vi "Compile Steps.vi"(8 "error in (no error)":errorcluster, 11 "Plugin in":refnum<class "Output Sequencer.lvclass">) -> (0 "error out":errorcluster, 3 "Plugin out":refnum<class "Output Sequencer.lvclass">)   [LabVIEW 2024, in "Output Sequencer.lvlib" / "Output Sequencer.lvclass"]
uses:
  Output Sequencer.lvclass
  Output Sequencer.lvclass/Output Sequencer.ctl
  Types/Expression Data.ctl
  <vilib>/LAVA/muParser/mupExpr/mupExpr.lvclass
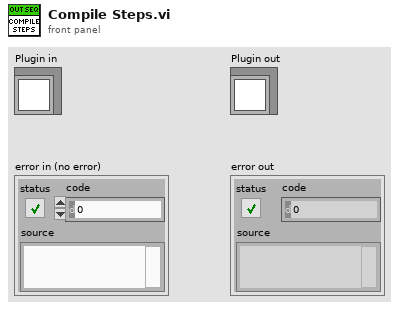
[diagram p1: front panel]
types:
  T1 = typedef "Output Sequencer.lvlib/Output Sequencer.lvclass/Expression Data.ctl" = cluster{"Empty?":bool, "Expression":refnum<class "mupExpr.lvclass">, "Variable Names":string[]}
  T2 = typedef "Output Sequencer.lvlib/Settings UI.lvclass/Step Settings.ctl" = cluster{"Description":string, "Precondition":string, "Duration":dbl, "Mode":string, "Delay Between Values":dbl, "Analog Values":string[], "Digital Values":string[], "Postcondition":string, "On True":string, "On False":string}
  T3 = typedef "Output Sequencer.lvlib/Output Sequencer.lvclass/Compiled Step.ctl" = cluster{"Precondition":T1, "Duration":dbl, "Mode":string, "Delay Between Values":dbl, "Analog Values":T1[], "Digital Values":T1[], "Postcondition":T1, "On True":string, "On False":string}
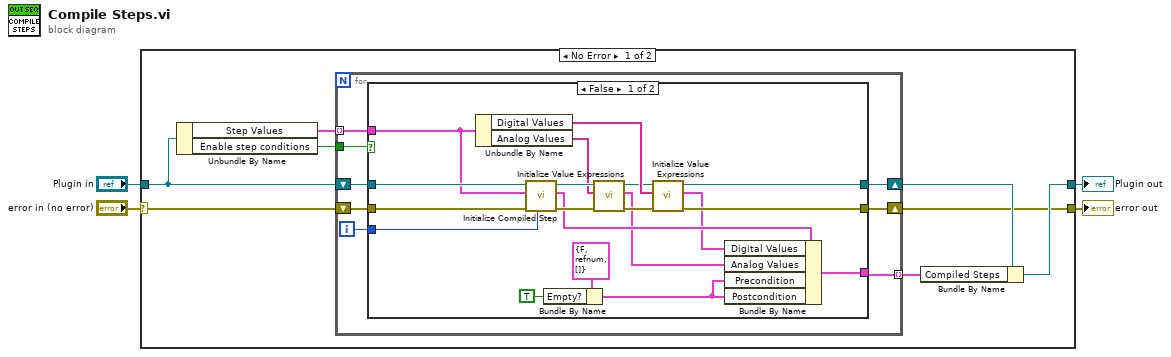
[diagram p0: block diagram]
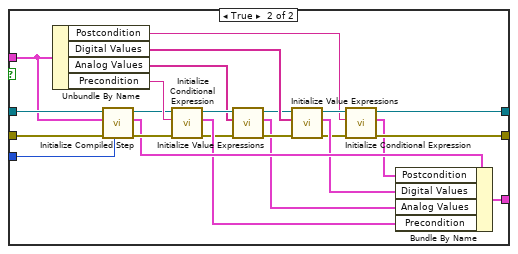
[diagram p2: hidden frame]
diagram:
  n1 = case shown="No Error" "error in (no error)" {
    selector: "error in (no error)" -> [w5 w65]
    tunnel: [w10 w64] -> w4
    tunnel: [w8 w65] -> w3
    tunnel: "Plugin in" -> [w7 w64]
    frame No Error {
      n2 = Unbundle By Name(w7) -> ("Step Values"=w12:T2[], "Enable step conditions"=w6:bool)
      n3 = for {
        tunnel: w12 -> [w18] mode=indexing
        tunnel: [w16] -> w11 mode=indexing
        shift-right: [w15] -> w9
        shift-left: w7 -> [w20]
        shift-right: [w17] -> w8
        shift-left: w5 -> [w19]
        tunnel: w6 -> [w14]
        i -> [w13]
        n4 = case shown="False" w14 {
          tunnel: w20 -> [w39 w63]
          tunnel: w19 -> [w38 w62]
          tunnel: w18 -> [w37 w61]
          tunnel: [w34 w57] -> w17
          tunnel: [w32 w53] -> w16
          tunnel: [w25 w42] -> w15
          tunnel: w13 -> [w21 w40]
          frame False {
            n5 = Unbundle By Name(w37) -> ("Digital Values"=w30:string[], "Analog Values"=w31:string[])
            n6 = call "Initialize Compiled Step.vi"("Step Number"=w21, "error in (no error)"=w38, "Step Values"=w37, "Output Sequencer in"=w39) -> ("error out"=w36:errorcluster, "Compiled Step"=w33:T3, "Output Sequencer out"=w35:refnum<class "Output Sequencer.lvclass">)  [unwired: 5 in]
            n7 = Bundle By Name(cluster=T1 {"Empty?"=FALSE, "Expression"=refnum, "Variable Names"=[]} ("Precondition"), "Empty?"=TRUE) -> (w22:T1)
            n8 = call "Initialize Value Expressions.vi"("error in (no error)"=w36, "Value strings"=w31, "Output Sequencer in"=w35) -> ("error out"=w28:errorcluster, "Expressions"=w27:T1[], "Output Sequencer out"=w29:refnum<class "Output Sequencer.lvclass">)  [unwired: 6 in]
            n9 = call "Initialize Value Expressions.vi"("error in (no error)"=w28, "Value strings"=w30, "Output Sequencer in"=w29) -> ("error out"=w34:errorcluster, "Expressions"=w26:T1[], "Output Sequencer out"=w25:refnum<class "Output Sequencer.lvclass">)  [unwired: 6 in]
            n10 = Bundle By Name(cluster=w33, "Digital Values"=w26, "Analog Values"=w27, "Precondition"=w22, "Postcondition"=w22) -> (w32:T3)
          }
          frame True {
            n11 = Unbundle By Name(w61) -> ("Postcondition"=w41:string, "Digital Values"=w49:string[], "Analog Values"=w50:string[], "Precondition"=w59:string)
            n12 = call "Initialize Compiled Step.vi"("Step Number"=w40, "error in (no error)"=w62, "Step Values"=w61, "Output Sequencer in"=w63) -> ("error out"=w60:errorcluster, "Compiled Step"=w56:T3, "Output Sequencer out"=w58:refnum<class "Output Sequencer.lvclass">)  [unwired: 5 in]
            n13 = call "Initialize Conditional Expression.vi"("error in (no error)"=w60, "Expression string"=w59, "Output Sequencer in"=w58) -> ("error out"=w51:errorcluster, "Expression Data"=w55:T1, "Output Sequencer out"=w52:refnum<class "Output Sequencer.lvclass">)  [unwired: 6 in]
            n14 = call "Initialize Value Expressions.vi"("error in (no error)"=w51, "Value strings"=w50, "Output Sequencer in"=w52) -> ("error out"=w47:errorcluster, "Expressions"=w46:T1[], "Output Sequencer out"=w48:refnum<class "Output Sequencer.lvclass">)  [unwired: 6 in]
            n15 = call "Initialize Value Expressions.vi"("error in (no error)"=w47, "Value strings"=w49, "Output Sequencer in"=w48) -> ("error out"=w44:errorcluster, "Expressions"=w45:T1[], "Output Sequencer out"=w43:refnum<class "Output Sequencer.lvclass">)  [unwired: 6 in]
            n16 = call "Initialize Conditional Expression.vi"("error in (no error)"=w44, "Expression string"=w41, "Output Sequencer in"=w43) -> ("error out"=w57:errorcluster, "Expression Data"=w54:T1, "Output Sequencer out"=w42:refnum<class "Output Sequencer.lvclass">)  [unwired: 6 in]
            n17 = Bundle By Name(cluster=w56, "Postcondition"=w54, "Digital Values"=w45, "Analog Values"=w46, "Precondition"=w55) -> (w53:T3)
          }
        }
      }
      n18 = Bundle By Name(cluster=w9, "Compiled Steps"=w11) -> (w10:refnum<class "Output Sequencer.lvclass">)
    }
    frame Error {
    }
  }
  "error out" <- w3
  "Plugin out" <- w4
